vi "asynchronous background process.vi"(10 "async data in":T1, 11 "module runtime in":refnum<class "TBM module execution interface.lvclass">) -> (0 "error out":errorcluster, 3 "module runtime out":refnum<class "TBM module execution interface.lvclass">)   [LabVIEW 2013, in "Standard Engine Runtime.lvclass"]
uses:
  Standard Engine Runtime.lvclass
  asynchronous process data.ctl
  <vilib>/NI/Tag Bus Module Framework/runtime/TBM module execution interface.lvclass
  async command notification.ctl
  <vilib>/NI/Tag Bus/table/data table.ctl
  <vilib>/NI/Tag Bus Module Framework/runtime/execution settings.ctl
  async error info.ctl
  <vilib>/NI/Tag Bus Module Framework/runtime/error classification.ctl
  <vilib>/NI/Tag Bus/table/data table.lvlib
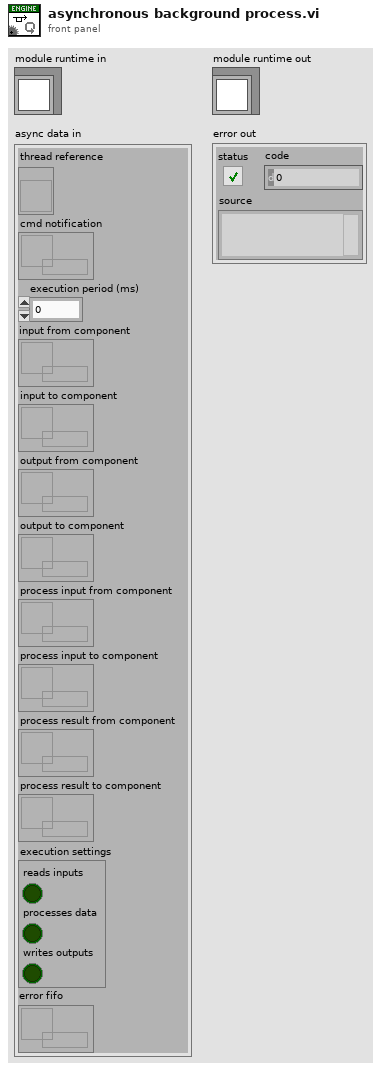
[diagram p1: front panel]
types:
  T1 = typedef "Standard Engine Runtime.lvclass/asynchronous process data.ctl" = cluster{"thread reference":refnum<vi>, "cmd notification":refnum<k33>, "execution period (ms)":i32, "input from component":refnum<queue>, "input to component":refnum<queue>, "output from component":refnum<queue>, "output to component":refnum<queue>, "process input from component":refnum<queue>, "process input to component":refnum<queue>, "process result from component":refnum<queue>, "process result to component":refnum<queue>, "execution settings":T2, "error fifo":refnum<k33>}
  T2 = typedef "TBM module execution interface.lvclass/execution settings.ctl" = cluster{"reads inputs":bool, "processes data":bool, "writes outputs":bool}
  T3 = typedef "TBM module execution interface.lvclass/error classification.ctl" = enum16{"unknown", "none", "trivial", "recoverable", "critical"}
  T4 = typedef "Standard Engine Runtime.lvclass/async error info.ctl" = cluster{"error code":i32, "error classification":T3}
  T5 = typedef "Standard Engine Runtime.lvclass/async command notification.ctl" = enum16{"stop", "safe state", "recover", "clear error"}
  T6 = typedef "tag bus.lvlib/data table.lvlib/data table.ctl" = cluster{"Double":dbl[], "Single":sgl[], "I64":i64[], "I32":i32[], "I16":i16[], "I8":i8[], "U64":u64[], "U32":u32[], "U16":u16[], "U8":u8[], "Boolean":bool[], "String":string[], "Array of Double":cluster{"DBL Array":dbl[]}[], "Array of Single":cluster{"SGL Array":sgl[]}[], "Array of I64":cluster{"I64 Array":i64[]}[], "Array of I32":cluster{"I32 Array":i32[]}[], "Array of I16":cluster{"I16 Array":i16[]}[], "Array of I8":cluster{"I8 Array":i8[]}[], "Array of U64":cluster{"U64 Array":u64[]}[], "Array of U32":cluster{"U32 Array":u32[]}[], "Array of U16":cluster{"U16 Array":u16[]}[], "Array of U8":cluster{"U8 Array":u8[]}[], "Array of Boolean":cluster{"Boolean Array":bool[]}[], "Array of String":cluster{"String Array":string[]}[]}
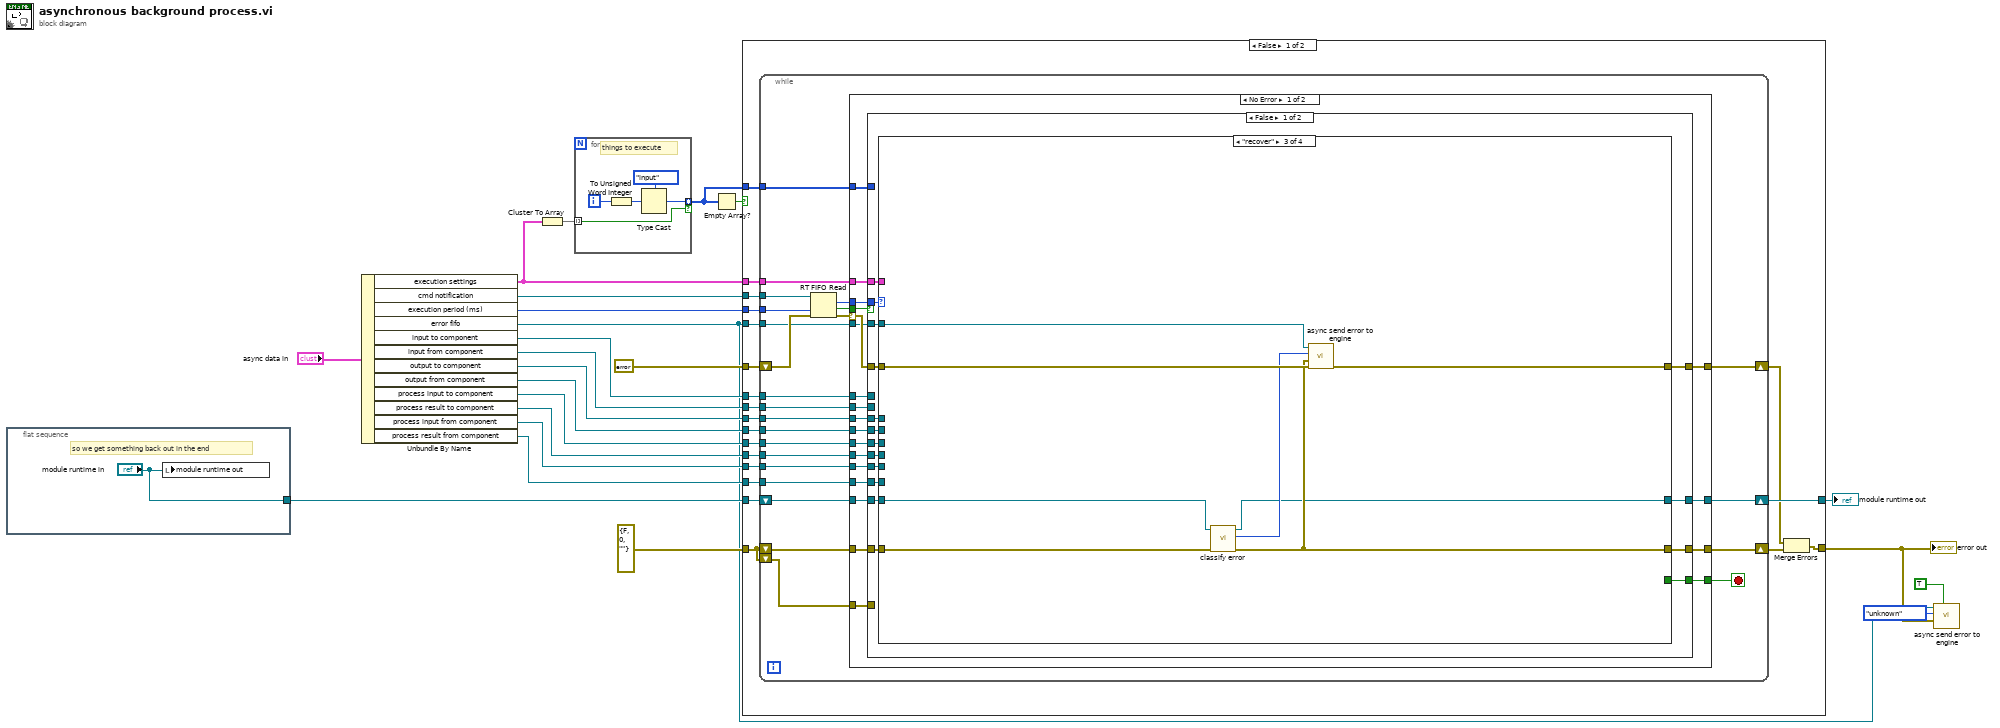
[diagram p0: block diagram]
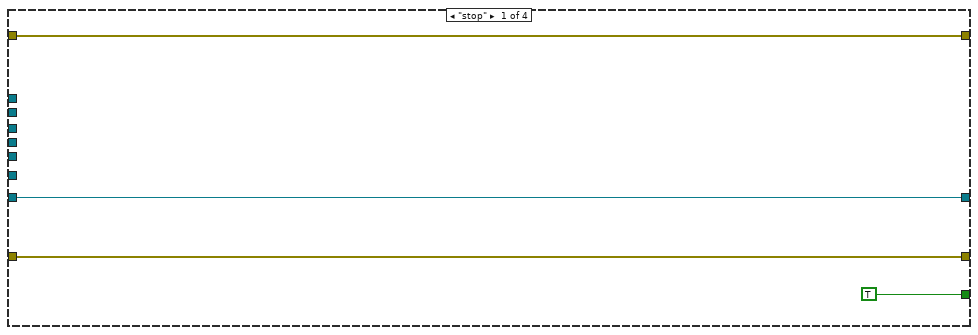
[diagram p2: hidden frame]
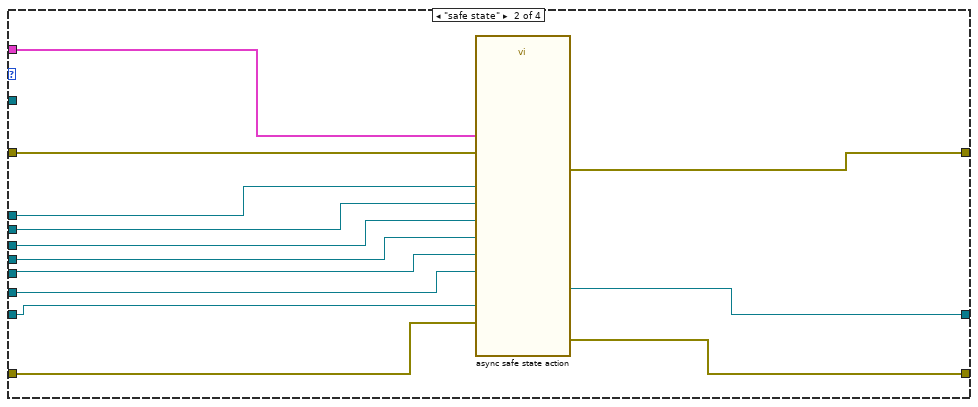
[diagram p3: hidden frame]
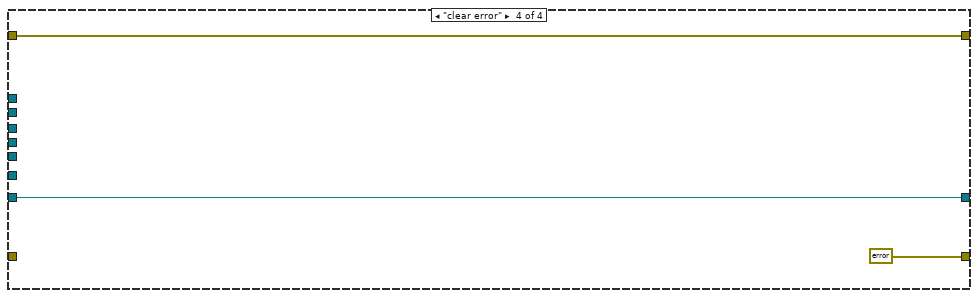
[diagram p4: hidden frame]
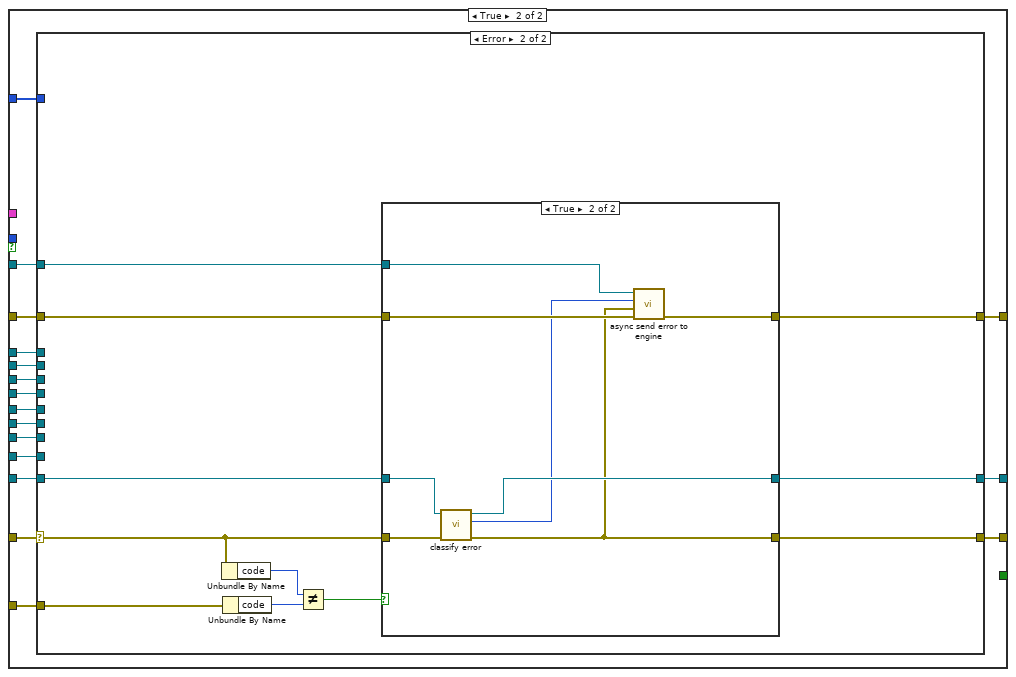
[diagram p5: hidden frame]
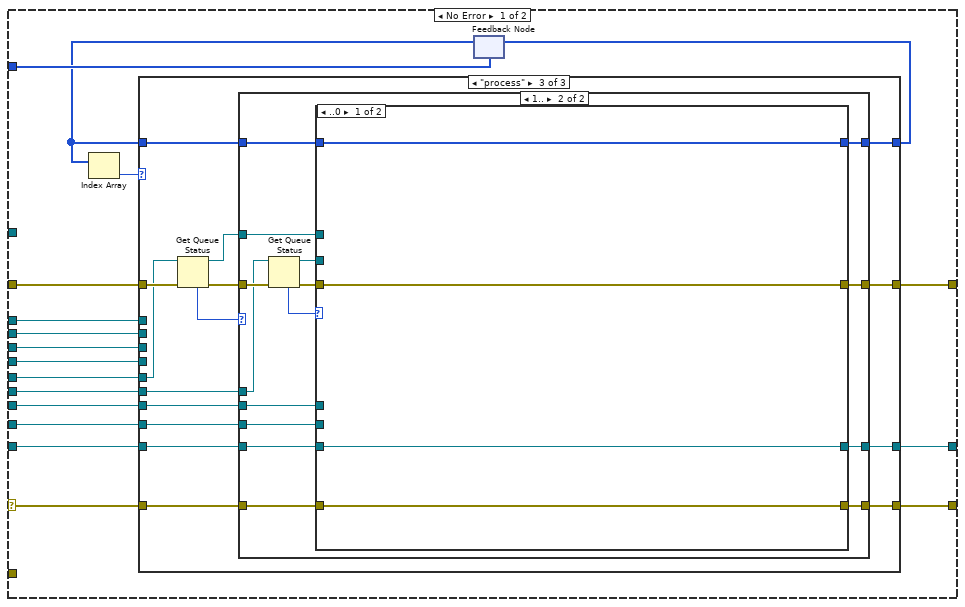
[diagram p6: hidden frame]
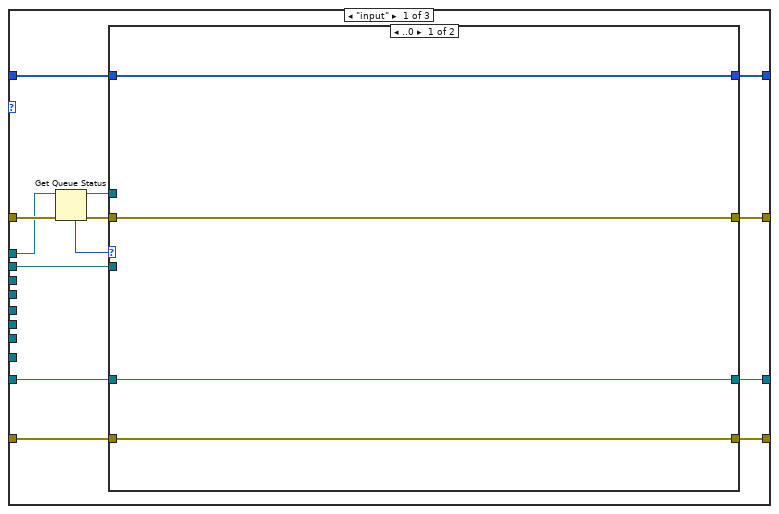
[diagram p7: hidden frame]
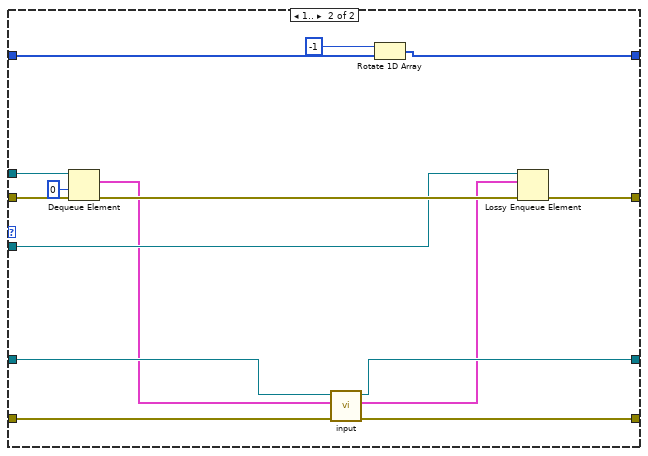
[diagram p8: hidden frame]
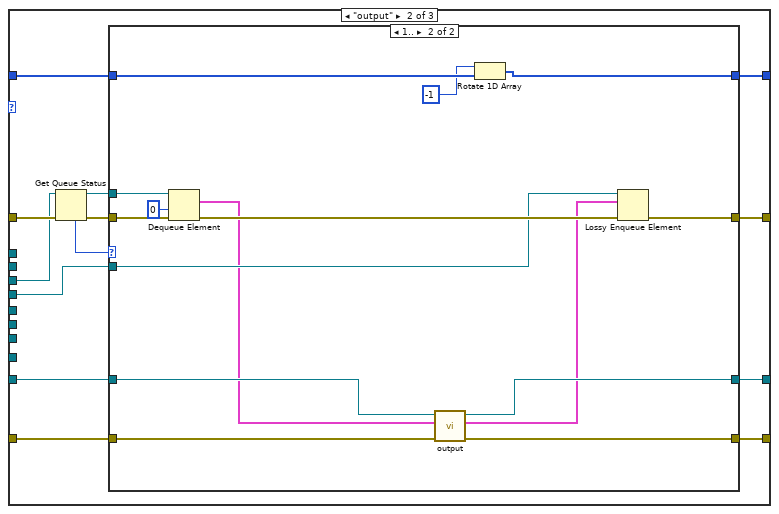
[diagram p9: hidden frame]
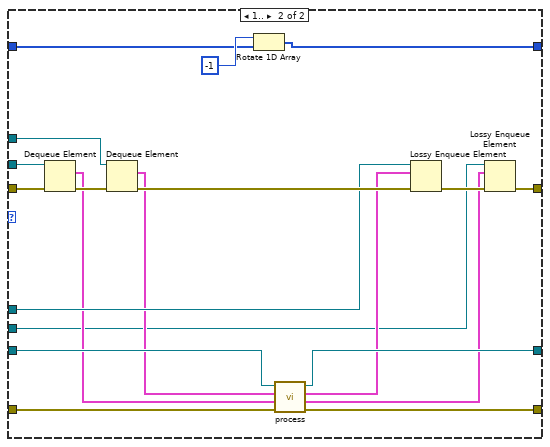
[diagram p12: hidden frame]
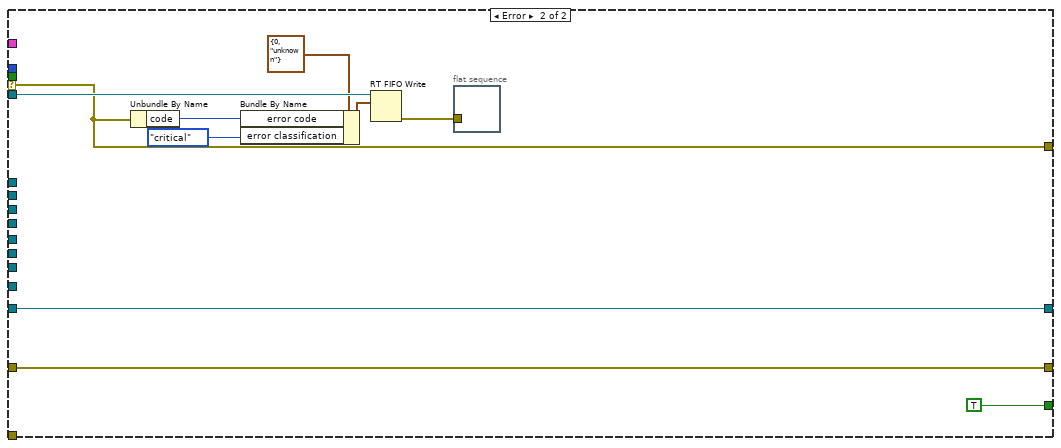
[diagram p14: hidden frame]
diagram:
  n1 = flat-sequence {
    tunnel: ["module runtime in"] -> w22
    frame #0 {
      # "so we get something back out in the end"
      n2 = local write "module runtime out"("module runtime in") -> ()
    }
  }
  n3 = Unbundle By Name("async data in") -> ("execution settings"=w2:T2, "cmd notification"=w20:refnum<k33>, "execution period (ms)"=w19:i32, "error fifo"=w5:refnum<k33>, "input to component"=w11:refnum<queue>, "input from component"=w10:refnum<queue>, "output to component"=w9:refnum<queue>, "output from component"=w12:refnum<queue>, "process input to component"=w13:refnum<queue>, "process result to component"=w14:refnum<queue>, "process input from component"=w15:refnum<queue>, "process result from component"=w16:refnum<queue>)
  n4 = Cluster To Array(cluster=w2) -> (array=w8:bool[])
  n5 = for {
    tunnel: w8 -> [w25] mode=indexing
    tunnel: [w26] -> w7 mode=indexing if=w25
    i -> [w27]
    # "things to execute"
    n6 = To Unsigned Word Integer(number=w27) -> (unsigned 16bit integer=w28:u16)
    n7 = Type Cast(type=enum16{"input", "process", "output"}."input" ("async execution state"), x=w28) -> (*(type *) &x=w26:enum16{"input", "process", "output"})
  }
  n8 = Empty Array?(array=w7) -> (empty?=w6:bool)
  n9 = case shown="False" w6 {
    tunnel: w22 -> [w49 w329]
    tunnel: [w48 w329] -> w21
    tunnel: w20 -> [w47 _]
    tunnel: w19 -> [w46 _]
    tunnel: errorcluster {"status"=FALSE, "code"=0, "source"=""} ("error out") -> [w30 w328]
    tunnel: [w43 w328] -> w4
    tunnel: w5 -> [w42 _]
    tunnel: errorcluster {"status"=FALSE, "code"=0, "source"=""} ("error out") -> [w41 _]
    tunnel: w16 -> [w40 _]
    tunnel: w15 -> [w39 _]
    tunnel: w14 -> [w38 _]
    tunnel: w13 -> [w37 _]
    tunnel: w12 -> [w36 _]
    tunnel: w11 -> [w35 _]
    tunnel: w10 -> [w34 _]
    tunnel: w9 -> [w33 _]
    tunnel: w7 -> [w32 _]
    tunnel: w2 -> [w31 _]
    frame False {
      n10 = while {
        shift-right: [w69] -> w48
        shift-left: w49 -> [w68]
        tunnel: w47 -> [w73]
        tunnel: w46 -> [w72]
        shift-right: [w66] -> w45
        shift-left: w30 -> [w51]
        shift-right: [w67] -> w44
        shift-left: w41 -> [w71]
        tunnel: w42 -> [w65]
        tunnel: w32 -> [w61]
        tunnel: w40 -> [w60]
        tunnel: w39 -> [w59]
        tunnel: w38 -> [w58]
        tunnel: w37 -> [w57]
        tunnel: w36 -> [w56]
        tunnel: w35 -> [w55]
        tunnel: w34 -> [w54]
        tunnel: w33 -> [w53]
        tunnel: w31 -> [w52]
        shift-left: w30 -> [w50]
        stop <- w64 stop-if-true
        n11 = RT FIFO Read(0:w73, 2:w72, 3:w71) -> (9:w63:T5, 10:w62:bool, 11:w70:errorcluster)  [unwired: 1 in, 2 out]
        n12 = case shown="No Error" w70 {
          selector: w70 -> [w89 w321]
          tunnel: [w91 w327] -> w69
          tunnel: w68 -> [w92 w327]
          tunnel: [w90 w321] -> w67
          tunnel: [w88 w326] -> w66
          tunnel: w51 -> [w76 w326]
          tunnel: w65 -> [w86 w325]
          tunnel: [w87 TRUE] -> w64
          tunnel: w63 -> [w93 _]
          tunnel: w62 -> [w94 _]
          tunnel: w61 -> [w85 _]
          tunnel: w60 -> [w84 _]
          tunnel: w59 -> [w83 _]
          tunnel: w58 -> [w82 _]
          tunnel: w57 -> [w81 _]
          tunnel: w56 -> [w80 _]
          tunnel: w55 -> [w79 _]
          tunnel: w54 -> [w78 _]
          tunnel: w53 -> [w77 _]
          tunnel: w52 -> [w75 _]
          tunnel: w50 -> [w74 _]
          frame No Error {
            n13 = case shown="False" w94 {
              tunnel: w93 -> [w110 _]
              tunnel: w92 -> [w109 w152]
              tunnel: [w108 w153] -> w91
              tunnel: [w107 w154] -> w90
              tunnel: w89 -> [w106 w155]
              tunnel: w76 -> [w105 w141]
              tunnel: [w104 w151] -> w88
              tunnel: [w103 _] -> w87
              tunnel: w86 -> [w102 w140]
              tunnel: w85 -> [_ w150]
              tunnel: w84 -> [w96 w149]
              tunnel: w83 -> [w97 w148]
              tunnel: w82 -> [w98 w147]
              tunnel: w81 -> [w99 w146]
              tunnel: w80 -> [w100 w145]
              tunnel: w79 -> [_ w144]
              tunnel: w78 -> [_ w143]
              tunnel: w77 -> [w101 w142]
              tunnel: w75 -> [w95 _]
              tunnel: w74 -> [_ w139]
              frame False {
                n14 = case shown="\"recover\"" w110 {
                  tunnel: w109 -> [w114 w123 w128 w137]
                  tunnel: [w114 w122 w129 w137] -> w108
                  tunnel: [w113 w126 w133 w138] -> w107
                  tunnel: w106 -> [w113 w127 w134 w138]
                  tunnel: w105 -> [w112 w124 w135 _]
                  tunnel: [w112 w121 w130 errorcluster {"status"=FALSE, "code"=0, "source"=""} ("classified error")] -> w104
                  tunnel: [TRUE _ _ _] -> w103
                  tunnel: w102 -> [_ _ w132 _]
                  tunnel: w101 -> [_ w115 _ _]
                  tunnel: w100 -> [_ w116 _ _]
                  tunnel: w99 -> [_ w117 _ _]
                  tunnel: w98 -> [_ w118 _ _]
                  tunnel: w97 -> [_ w119 _ _]
                  tunnel: w96 -> [_ w120 _ _]
                  tunnel: w95 -> [_ w125 _ _]
                  frame "stop" {
                  }
                  frame "safe state" {
                    n15 = call "async safe state action.vi"("output to component"=w115, "system error in"=w127, "execution settings"=w125, "output from component"=w116, "process input to component"=w117, "process result to component"=w118, "process input from component"=w119, "process result from component"=w120, "module in"=w123, "module error in"=w124) -> ("system error out"=w126:errorcluster, "module out"=w122:refnum<class "TBM module execution interface.lvclass">, "module error out"=w121:errorcluster)  [unwired: 3 in]
                  }
                  frame "recover" {
                    n16 = call-dynamic "classify error.vi"("error to classify"=w135, "module in"=w128) -> ("classified error"=w130:errorcluster, "error classification"=w131:T3, "module out"=w129:refnum<class "TBM module execution interface.lvclass">)  [unwired: 7 in]
                    n17 = call "async send error to engine.vi"("command error in"=w134, "module error"=w130, "error classification"=w131, "error fifo"=w132) -> ("command error out"=w133:errorcluster)  [unwired: 7 in]
                  }
                  frame "clear error" {
                  }
                }
              }
              frame True {
                n18 = case shown="Error" w141 {
                  selector: w141 -> [w157 w297]
                  tunnel: w155 -> [w172 w306]
                  tunnel: [w171 w304] -> w154
                  tunnel: [w170 w303] -> w153
                  tunnel: w152 -> [w169 w302]
                  tunnel: [w156 w301] -> w151
                  tunnel: w150 -> [w168 _]
                  tunnel: w149 -> [w167 _]
                  tunnel: w148 -> [w166 _]
                  tunnel: w147 -> [w165 _]
                  tunnel: w146 -> [w164 _]
                  tunnel: w145 -> [w163 _]
                  tunnel: w144 -> [w162 _]
                  tunnel: w143 -> [w161 _]
                  tunnel: w142 -> [w160 _]
                  tunnel: w140 -> [_ w305]
                  tunnel: w139 -> [_ w296]
                  frame No Error {
                    n19 = feedback #1(w168) -> (w158:enum16{"input", "process", "output"}[])
                    n20 = Index Array(array=w158) -> (element=w159:enum16{"input", "process", "output"})  [unwired: 1 in]
                    n21 = case shown="\"process\"" w159 {
                      tunnel: [w181 w214 w248] -> w173
                      tunnel: w172 -> [w186 w218 w252]
                      tunnel: [w180 w213 w247] -> w171
                      tunnel: [w179 w212 w246] -> w170
                      tunnel: w169 -> [w178 w211 w245]
                      tunnel: w157 -> [w177 w210 w244]
                      tunnel: [w176 w209 w243] -> w156
                      tunnel: w167 -> [_ _ w238]
                      tunnel: w166 -> [_ _ w239]
                      tunnel: w165 -> [_ _ w240]
                      tunnel: w164 -> [_ _ w241]
                      tunnel: w163 -> [_ w206 _]
                      tunnel: w162 -> [w185 _ _]
                      tunnel: w161 -> [w174 _ _]
                      tunnel: w160 -> [_ w207 _]
                      tunnel: w158 -> [w175 w208 w242]
                      frame "input" {
                        n22 = Get Queue Status(queue=w185, error in (no error)=w186) -> (queue out=w182:refnum<queue>, error out=w183:errorcluster, # elements in queue=w184:i32)  [unwired: 1 in, 5 out]
                        n23 = case shown="..0" w184 {
                          tunnel: w183 -> [w190 w204]
                          tunnel: w182 -> [_ w205]
                          tunnel: [w187 w194] -> w181
                          tunnel: [w190 w197] -> w180
                          tunnel: [w189 w199] -> w179
                          tunnel: w178 -> [w189 w201]
                          tunnel: w177 -> [w188 w202]
                          tunnel: [w188 w200] -> w176
                          tunnel: w175 -> [w187 w193]
                          tunnel: w174 -> [_ w196]
                          frame ..0 {
                          }
                          frame 1.. {
                            n24 = Dequeue Element(queue=w205, timeout in ms (-1)=0, error in (no error)=w204) -> (element=w195:T6, error out=w198:errorcluster)  [unwired: 2 out]
                            n25 = call-dynamic "input.vi"("error in"=w202, "input allocation"=w195, "module in"=w201) -> ("error out"=w200:errorcluster, "input data"=w192:T6, "module out"=w199:refnum<class "TBM module execution interface.lvclass">)  [unwired: 6 in]
                            n26 = Rotate 1D Array(1:w193, 2:-1 ("n")) -> (0:w194:enum16{"input", "process", "output"}[])
                            n27 = Lossy Enqueue Element(queue=w196, element=w192, error in (no error)=w198) -> (error out=w197:errorcluster)  [unwired: 3 out]
                          }
                        }
                      }
                      frame "output" {
                        n28 = Get Queue Status(queue=w207, error in (no error)=w218) -> (queue out=w215:refnum<queue>, error out=w216:errorcluster, # elements in queue=w217:i32)  [unwired: 1 in, 5 out]
                        n29 = case shown="1.." w217 {
                          tunnel: w216 -> [w222 w236]
                          tunnel: w215 -> [_ w237]
                          tunnel: [w219 w226] -> w214
                          tunnel: [w222 w229] -> w213
                          tunnel: [w221 w231] -> w212
                          tunnel: w211 -> [w221 w233]
                          tunnel: w210 -> [w220 w234]
                          tunnel: [w220 w232] -> w209
                          tunnel: w208 -> [w219 w225]
                          tunnel: w206 -> [_ w228]
                          frame ..0 {
                          }
                          frame 1.. {
                            n30 = Dequeue Element(queue=w237, timeout in ms (-1)=0, error in (no error)=w236) -> (element=w227:T6, error out=w230:errorcluster)  [unwired: 2 out]
                            n31 = call-dynamic "output.vi"("error in"=w234, "output data"=w227, "module in"=w233) -> ("error out"=w232:errorcluster, "output allocation"=w223:T6, "module out"=w231:refnum<class "TBM module execution interface.lvclass">)  [unwired: 6 in]
                            n32 = Rotate 1D Array(1:w225, 2:-1 ("n")) -> (0:w226:enum16{"input", "process", "output"}[])
                            n33 = Lossy Enqueue Element(queue=w228, element=w223, error in (no error)=w230) -> (error out=w229:errorcluster)  [unwired: 3 out]
                          }
                        }
                      }
                      frame "process" {
                        n34 = Get Queue Status(queue=w241, error in (no error)=w252) -> (queue out=w249:refnum<queue>, error out=w250:errorcluster, # elements in queue=w251:i32)  [unwired: 1 in, 5 out]
                        n35 = case shown="1.." w251 {
                          tunnel: w250 -> [w256 w271]
                          tunnel: w249 -> [_ w259]
                          tunnel: [w253 w267] -> w248
                          tunnel: [w256 w265] -> w247
                          tunnel: [w255 w262] -> w246
                          tunnel: w245 -> [w255 w263]
                          tunnel: w244 -> [w254 w261]
                          tunnel: [w254 w260] -> w243
                          tunnel: w242 -> [w253 w266]
                          tunnel: w240 -> [_ w270]
                          tunnel: w239 -> [_ w258]
                          tunnel: w238 -> [_ w257]
                          frame ..0 {
                          }
                          frame 1.. {
                            n36 = Get Queue Status(queue=w270, error in (no error)=w271) -> (queue out=w264:refnum<queue>, error out=w268:errorcluster, # elements in queue=w269:i32)  [unwired: 1 in, 5 out]
                            n37 = case shown="..0" w269 {
                              tunnel: w268 -> [w274 w295]
                              tunnel: [w275 w289] -> w267
                              tunnel: w266 -> [w275 w290]
                              tunnel: [w274 w288] -> w265
                              tunnel: w264 -> [_ w294]
                              tunnel: w263 -> [w273 w284]
                              tunnel: [w273 w283] -> w262
                              tunnel: w261 -> [w272 w285]
                              tunnel: [w272 w282] -> w260
                              tunnel: w259 -> [_ w292]
                              tunnel: w258 -> [_ w281]
                              tunnel: w257 -> [_ w277]
                              frame ..0 {
                              }
                              frame 1.. {
                                n38 = Dequeue Element(queue=w294, error in (no error)=w295) -> (element=w280:T6, error out=w293:errorcluster)  [unwired: 1 in, 2 out]
                                n39 = Dequeue Element(queue=w292, error in (no error)=w293) -> (element=w279:T6, error out=w286:errorcluster)  [unwired: 1 in, 2 out]
                                n40 = Rotate 1D Array(1:w290, 2:-1 ("n")) -> (0:w289:enum16{"input", "process", "output"}[])
                                n41 = call-dynamic "process.vi"("error in"=w285, "result allocation"=w280, "parameters"=w279, "module in"=w284) -> ("error out"=w282:errorcluster, "results"=w276:T6, "parameter allocation"=w278:T6, "module out"=w283:refnum<class "TBM module execution interface.lvclass">)  [unwired: 4 in]
                                n42 = Lossy Enqueue Element(queue=w281, element=w278, error in (no error)=w286) -> (error out=w287:errorcluster)  [unwired: 3 out]
                                n43 = Lossy Enqueue Element(queue=w277, element=w276, error in (no error)=w287) -> (error out=w288:errorcluster)  [unwired: 3 out]
                              }
                            }
                          }
                        }
                      }
                    }
                    n44 = feedback-in #1(w173) -> ()
                  }
                  frame Error {
                    n45 = Unbundle By Name(w297) -> ("code"=w299:i32)
                    n46 = Unbundle By Name(w296) -> ("code"=w300:i32)
                    n47 = Not Equal?(x=w299, y=w300) -> (x != y?=w298:bool)
                    n48 = case shown="True" w298 {
                      tunnel: w306 -> [w309 w317]
                      tunnel: w305 -> [_ w316]
                      tunnel: [w309 w315] -> w304
                      tunnel: [w308 w314] -> w303
                      tunnel: w302 -> [w308 w313]
                      tunnel: [w307 w311] -> w301
                      tunnel: w297 -> [w307 w310]
                      frame False {
                      }
                      frame True {
                        n49 = call-dynamic "classify error.vi"("error to classify"=w310, "module in"=w313) -> ("classified error"=w311:errorcluster, "error classification"=w312:T3, "module out"=w314:refnum<class "TBM module execution interface.lvclass">)  [unwired: 7 in]
                        n50 = call "async send error to engine.vi"("command error in"=w317, "module error"=w311, "error classification"=w312, "error fifo"=w316) -> ("command error out"=w315:errorcluster)  [unwired: 7 in]
                      }
                    }
                  }
                }
              }
            }
          }
          frame Error {
            n51 = Unbundle By Name(w321) -> ("code"=w320:i32)
            n52 = Bundle By Name(cluster=T4 {"error code"=0, "error classification"=enum."unknown"} ("element"), "error code"=w320, "error classification"=error_classification."critical") -> (w322:T4)
            n53 = RT FIFO Write(0:w325, 1:w322) -> (11:w324:errorcluster)  [unwired: 3 in, 3 out]
            n54 = flat-sequence {
              tunnel: w324 -> [_]
              frame #0 {
              }
            }
          }
        }
      }
      n55 = Merge Errors(w44, w45) -> (w43:errorcluster)
    }
    frame True {
    }
  }
  "error out" <- w4
  "module runtime out" <- w21
  n56 = call "async send error to engine.vi"("force send?"=TRUE, "module error"=w4, "error classification"=error_classification."unknown", "error fifo"=w5) -> ()  [unwired: 7 in, 1 out]
